vi "Bundle Script_Named (Un)Bundler Reorder.vi"(4 "Hide Full Names":bool=TRUE, 5 "Ignore Hide Full Names":bool=TRUE, 8 "error in":errorcluster, 10 "Displayed Items":string[](array[string]), 11 "Affected Items":T1) -> (0 "error out":errorcluster, 2 "Objects":refnum<vi>[](array[refnum]))   [LabVIEW 2023]
doc: "Tag tree tags as input, as these contain the original indices, which are used for reordering the wires and labels of the bundle or unbundle by name structures"
uses:
  top/BundleMagic.ctl
panel:
  out "Array":cluster{"Array":bool[]}[](array[cluster])
  out "Bundle Type":T2(ring)
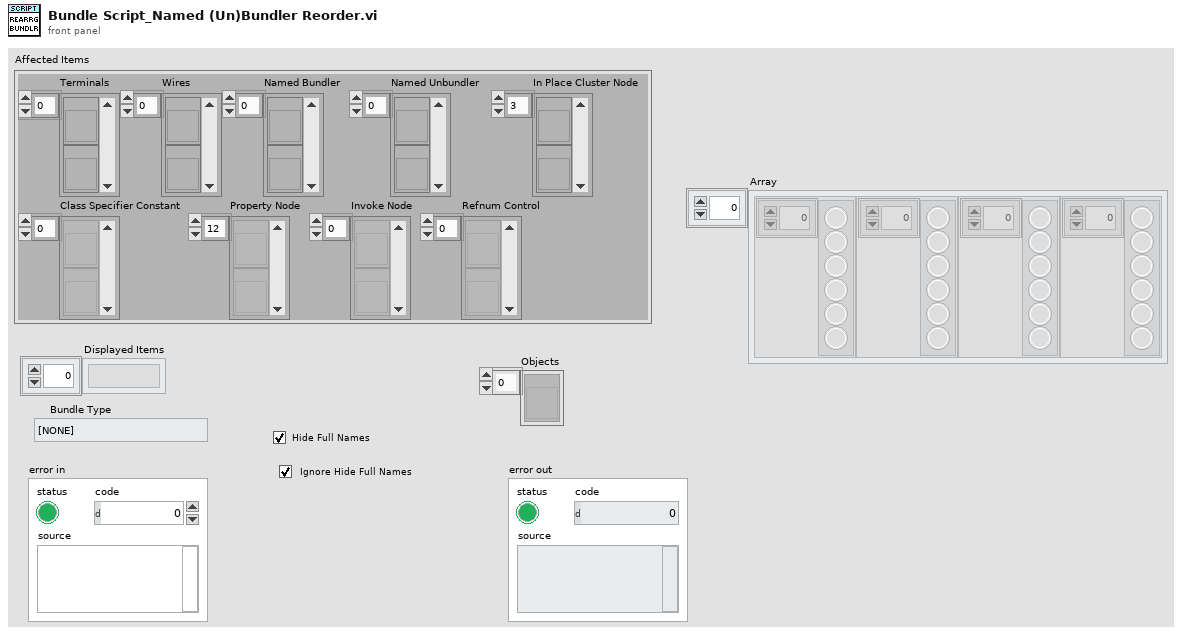
[diagram p1: front panel]
types:
  T1 = typedef "BundleMagic.ctl" = cluster{"Terminals":refnum<vi>[], "Wires":refnum<vi>[], "Named Bundler":refnum<vi>[], "Named Unbundler":refnum<vi>[], "In Place Cluster Node":refnum<vi>[], "Class Specifier Constant":refnum<vi>[], "Property Node":refnum<vi>[], "Invoke Node":refnum<vi>[], "Refnum Control":refnum<vi>[]}
  T2 = enum16{"[NONE]", "Unbundle", "Bundle", "Insert Before", "Insert After", "Remove Elements", "Rearrange Elements"}
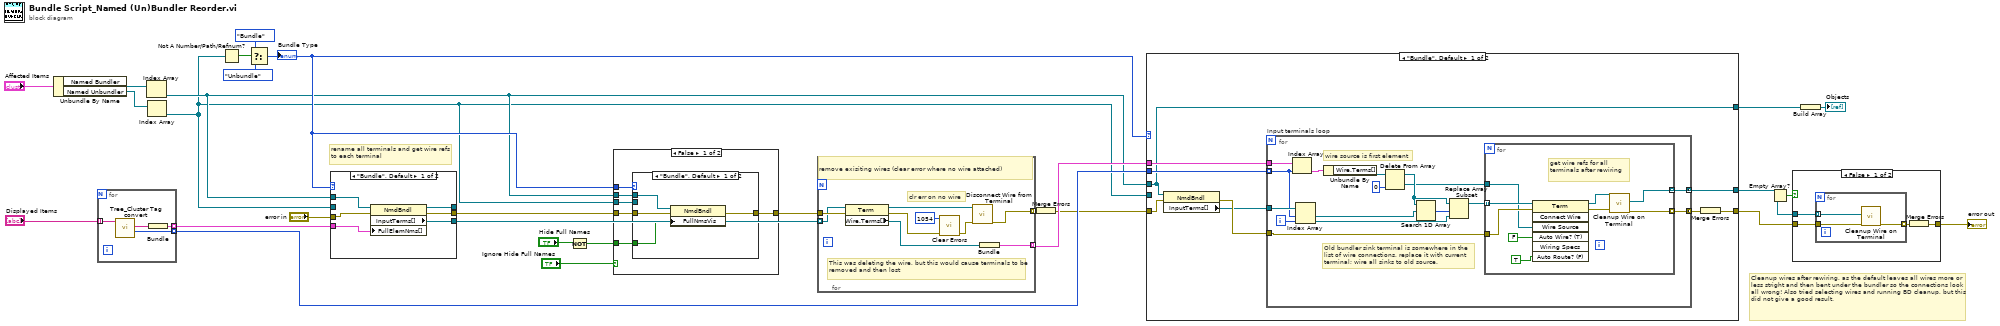
[diagram p0: block diagram]
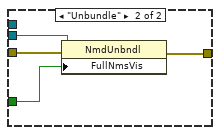
[diagram p2: hidden frame]
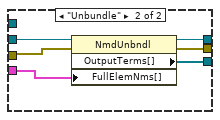
[diagram p4: hidden frame]
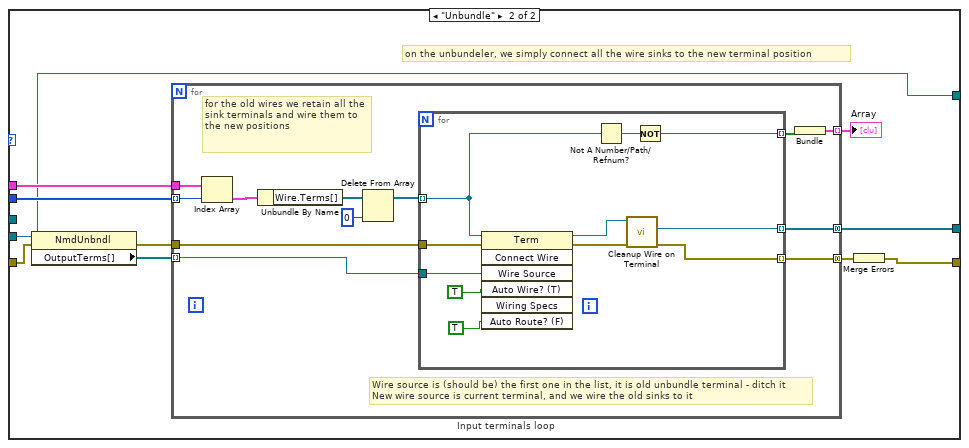
[diagram p5: hidden frame]
diagram:
  # "Cleanup wires after rewiring, as the default leaves all wires more or less stright and then bent under the bundler so the connections look all wrong! Also tried selecting wires and running BD cleanup, but this did not give a good result."
  # "rename all terminals and get wire refs to each terminal"
  n1 = Unbundle By Name("Affected Items") -> ("Named Bundler"=w20:refnum<vi>[], "Named Unbundler"=w18:refnum<vi>[])
  n2 = for {
    tunnel: "Displayed Items" -> [w32] mode=indexing
    tunnel: [w29] -> w22 mode=indexing
    tunnel: [w30] -> w24 mode=indexing
    n3 = call "Tree_Cluster Tag convert.vi"("Tag"=w32) -> ("Index"=w30:u32, "Tree Nest"=w31:string[])  [unwired: 5 in, 4 out]
    n4 = Bundle("Tree Nest"=w31) -> (w29:cluster{"Tree Nest":string[]})  [unwired: 1 in]
  }
  n5 = Index Array(array=w20) -> (element=w6:refnum<vi>)  [unwired: 1 in]
  n6 = Index Array(array=w18) -> (element=w5:refnum<vi>)  [unwired: 1 in]
  n7 = Not A Number/Path/Refnum?(number/path/refnum=w5) -> (NaN/Path/Refnum?=w17:bool)
  n8 = Select(t=T2."Bundle" ("Action"), s=w17, f=T2."Unbundle" ("Action")) -> (s? t:f=w7:T2)
  "Bundle Type" <- w7
  n9 = case shown="\"Bundle\", Default" w7 {
    tunnel: [w35 w44] -> w26
    tunnel: [w36 w43] -> w4
    tunnel: w6 -> [w38 _]
    tunnel: w22 -> [w37 w41]
    tunnel: w5 -> [_ w42]
    tunnel: "error in" -> [w34 w40]
    tunnel: [w33 w39] -> _
    frame "Bundle", Default {
      n10 = property class="NmdBndl"(reference=w38, error in=w34, "FullElemNms[]"=w37) -> (reference out=w33:refnum<vi>, error out=w36:errorcluster, "InputTerms[]"=w35:refnum<vi>[])
    }
    frame "Unbundle" {
      n11 = property class="NmdUnbndl"(reference=w42, error in=w40, "FullElemNms[]"=w41) -> (reference out=w39:refnum<vi>, error out=w43:errorcluster, "OutputTerms[]"=w44:refnum<vi>[])
    }
  }
  n12 = Not(x="Hide Full Names") -> (.not. x?=w2:bool)
  n13 = case shown="False" "Ignore Hide Full Names" {
    tunnel: w7 -> [w50 _]
    tunnel: w6 -> [w49 _]
    tunnel: w5 -> [w48 _]
    tunnel: w4 -> [w47 w59]
    tunnel: [w46 w59] -> w3
    tunnel: w2 -> [w45 _]
    frame False {
      n14 = case shown="\"Bundle\", Default" w50 {
        tunnel: [w54 w58] -> w46
        tunnel: w49 -> [w52 _]
        tunnel: w48 -> [_ w57]
        tunnel: w47 -> [w53 w56]
        tunnel: w45 -> [w51 w55]
        frame "Bundle", Default {
          n15 = property class="NmdBndl"(reference=w52, error in=w53, "FullNmsVis"=w51) -> (error out=w54:errorcluster)  [unwired: 1 out]
        }
        frame "Unbundle" {
          n16 = property class="NmdUnbndl"(reference=w57, error in=w56, "FullNmsVis"=w55) -> (error out=w58:errorcluster)  [unwired: 1 out]
        }
      }
    }
    frame True {
    }
  }
  n17 = for {
    tunnel: w26 -> [w67] mode=indexing
    tunnel: [w65] -> w25 mode=indexing
    tunnel: w3 -> [w68]
    tunnel: [w62] -> w23 mode=indexing
    # "This was deleting the wire, but this would cause terminals to be removed and then lost"
    # "clr err on no wire"
    # "remove exisiting wires (clear error where no wire attached)"
    n18 = property class="Term"(reference=w67, error in=w68) -> (reference out=w64:refnum<vi>, error out=w63:errorcluster, "Wire.Terms[]"=w66:refnum<vi>[])
    n19 = call <vilib>:"Clear Errors.vi"("error in (no error)"=w63, "specific error code to clear (0: all)"=1054) -> ("error out"=w61:errorcluster)  [unwired: 4 in, 1 out]
    n20 = call "Disconnect Wire from Terminal.vi"("error in"=w61, "Terminal in"=w64) -> ("error out"=w62:errorcluster)  [unwired: 5 in, 4 out]
    n21 = Bundle("Wire.Terms[]"=w66) -> (w65:cluster{"Wire.Terms[]":refnum<vi>[]})  [unwired: 1 in]
  }
  n22 = Merge Errors(w23) -> (w9:errorcluster)
  n23 = case shown="\"Bundle\", Default" w7 {
    tunnel: w9 -> [w74 w109]
    tunnel: w25 -> [w76 w111]
    tunnel: w6 -> [w70 _]
    tunnel: w5 -> [_ w104]
    tunnel: w24 -> [w73 w108]
    tunnel: [w72 w106] -> w11
    tunnel: [w69 w103] -> w16
    tunnel: [w70 w104] -> w13
    frame "Bundle", Default {
      n24 = property class="NmdBndl"(reference=w70, error in=w74) -> (error out=w77:errorcluster, "InputTerms[]"=w75:refnum<vi>[])  [unwired: 1 out]
      n25 = for "Input terminals loop" {
        tunnel: w76 -> [w92]
        tunnel: w73 -> [w89] mode=indexing
        tunnel: w75 -> [w90]
        tunnel: w77 -> [w93]
        tunnel: [w79] -> w72 mode=concatenating
        tunnel: [w78] -> w71 mode=concatenating
        i -> [w88]
        # "wire source is first element"
        # "Old bundler sink terminal is somewhere in the list of wire connections, replace it with current terminal; wire all sinks to old source."
        n26 = Index Array(array=w92, index=w89) -> (element=w91:cluster{"Wire.Terms[]":refnum<vi>[]})
        n27 = Index Array(array=w90, index #1=w89, index #2=w88) -> (element #1=w86:refnum<vi>, element #2=w84:refnum<vi>)
        n28 = Unbundle By Name(w91) -> ("Wire.Terms[]"=w87:refnum<vi>[])
        n29 = Delete From Array(array=w87, index=0) -> (deleted portion=w80:refnum<vi>, array with subset deleted=w82:refnum<vi>[])  [unwired: 1 in]
        n30 = Search 1D Array(1D array=w82, element=w86) -> (index of element=w85:i32)  [unwired: 1 in]
        n31 = Replace Array Subset(array=w82, new element=w84, index=w85) -> (w83:refnum<vi>[])
        n32 = for {
          tunnel: w93 -> [w102]
          tunnel: w83 -> [w101] mode=indexing
          tunnel: w80 -> [w99]
          tunnel: [w95] -> w79 mode=indexing
          tunnel: [w94] -> w78 mode=indexing
          # "get wire refs for all terminals after rewiring"
          n33 = invoke class="Term" method="Connect Wire"(reference=w101, error in=w102, "Wire Source"=w99, "Auto Wire? (T)"=FALSE, "Auto Route? (F)"=TRUE) -> (reference out=w96:refnum<vi>, error out=w97:errorcluster)  [unwired: 2 in, 5 out]
          n34 = call "Cleanup Wire on Terminal.vi"("error in"=w97, "Terminal in"=w96) -> ("error out"=w94:errorcluster, "Wire out"=w95:refnum<vi>)  [unwired: 7 in, 1 out]
        }
      }
      n35 = Merge Errors(w71) -> (w69:errorcluster)
    }
    frame "Unbundle" {
      # "on the unbundeler, we simply connect all the wire sinks to the new terminal position"
      n36 = property class="NmdUnbndl"(reference=w104, error in=w109) -> (error out=w112:errorcluster, "OutputTerms[]"=w110:refnum<vi>[])  [unwired: 1 out]
      n37 = for "Input terminals loop" {
        tunnel: w111 -> [w121]
        tunnel: w108 -> [w119] mode=indexing
        tunnel: w112 -> [w124]
        tunnel: w110 -> [w122] mode=indexing
        tunnel: [w117] -> w106 mode=concatenating
        tunnel: [w116] -> w107 mode=concatenating
        tunnel: [w113] -> w105 mode=indexing
        # "for the old wires we retain all the sink terminals and wire them to the new positions"
        # "Wire source is (should be) the first one in the list, it is old unbundle terminal - ditch it\nNew wire source is current terminal, and we wire the old sinks to it"
        n38 = Index Array(array=w121, index=w119) -> (element=w120:cluster{"Wire.Terms[]":refnum<vi>[]})
        n39 = Unbundle By Name(w120) -> ("Wire.Terms[]"=w123:refnum<vi>[])
        n40 = Delete From Array(array=w123, index=0) -> (array with subset deleted=w115:refnum<vi>[])  [unwired: 1 in, 1 out]
        n41 = for {
          tunnel: w124 -> [w135]
          tunnel: w115 -> [w131] mode=indexing
          tunnel: w122 -> [w133]
          tunnel: [w128] -> w117 mode=indexing
          tunnel: [w126] -> w116 mode=indexing
          tunnel: [w129] -> w114 mode=indexing
          n42 = invoke class="Term" method="Connect Wire"(reference=w131, error in=w135, "Wire Source"=w133, "Auto Wire? (T)"=TRUE ("Auto Route? (F)"), "Auto Route? (F)"=TRUE) -> (reference out=w125:refnum<vi>, error out=w127:errorcluster)  [unwired: 2 in, 5 out]
          n43 = Not A Number/Path/Refnum?(number/path/refnum=w131) -> (NaN/Path/Refnum?=w130:bool)
          n44 = call "Cleanup Wire on Terminal.vi"("error in"=w127, "Terminal in"=w125) -> ("error out"=w126:errorcluster, "Wire out"=w128:refnum<vi>)  [unwired: 7 in, 1 out]
          n45 = Not(x=w130) -> (.not. x?=w129:bool)
        }
        n46 = Bundle(w114) -> (w113:cluster{bool[]})  [unwired: 1 in]
      }
      "Array" <- w105
      n47 = Merge Errors(w107) -> (w103:errorcluster)
    }
  }
  n48 = Empty Array?(array=w11) -> (empty?=w10:bool)
  n49 = case shown="False" w10 {
    tunnel: w11 -> [w139 _]
    tunnel: w16 -> [w138 w143]
    tunnel: [w136 w143] -> w15
    frame False {
      n50 = for {
        tunnel: w139 -> [w140] mode=indexing
        tunnel: w138 -> [w142]
        tunnel: [w141] -> w137 mode=indexing
        n51 = call "Cleanup Wire on Terminal.vi"("error in"=w142, "Wire In"=w140) -> ("error out"=w141:errorcluster)  [unwired: 7 in, 2 out]
      }
      n52 = Merge Errors(w137) -> (w136:errorcluster)
    }
    frame True {
    }
  }
  "error out" <- w15
  n53 = Build Array(w13) -> (→"Objects":refnum<vi>[])
